vi "Get Encoders.vi"   [LabVIEW 2012]
uses:
  Robot Global Data.vi
types:
  T1 = typedef "WPI_EncoderDevRef.ctl" = cluster{"DevStatus":errorcluster, "EncoderIndex":T2, "CounterIndex":T3, "DistancePerCount":dbl, "Decoding Type":T4}
  T2 = typedef "FPGA_EncoderIdx.ctl" = enum8{"Enc 0", "Enc 1", "Enc 2", "Enc 3", "Invalid"}
  T3 = typedef "FPGA_CounterCtrSystemIndex.ctl" = enum8{"Ctr 0", "Ctr 1", "Ctr 2", "Ctr 3", "Ctr 4", "Ctr 5", "Ctr 6", "Ctr 7", "Invalid"}
  T4 = typedef "WPI_EncoderType.ctl" = enum16{"1x", "2x", "4x"}
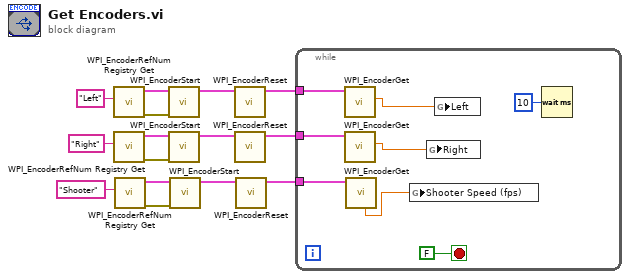
[diagram p0: block diagram]
diagram:
  n1 = call <vilib>:"WPI_EncoderRefNum Registry Get.vi"("refnum name"="Left") -> ("error out"=w15:errorcluster, "EncoderDevRef"=w14:T1)  [unwired: 9 in]
  n2 = call <vilib>:"WPI_EncoderRefNum Registry Get.vi"("refnum name"="Right") -> ("error out"=w10:errorcluster, "EncoderDevRef"=w9:T1)  [unwired: 9 in]
  n3 = call <vilib>:"WPI_EncoderRefNum Registry Get.vi"("refnum name"="Shooter") -> ("error out"=w5:errorcluster, "EncoderDevRef"=w4:T1)  [unwired: 9 in]
  n4 = call <vilib>:"WPI_EncoderStart.vi"("error in (no error)"=w15, "EncoderDevRef"=w14) -> ("EncoderDevRef"=w13:T1)  [unwired: 8 in, 1 out]
  n5 = call <vilib>:"WPI_EncoderStart.vi"("error in (no error)"=w10, "EncoderDevRef"=w9) -> ("EncoderDevRef"=w8:T1)  [unwired: 8 in, 1 out]
  n6 = call <vilib>:"WPI_EncoderStart.vi"("error in (no error)"=w5, "EncoderDevRef"=w4) -> ("EncoderDevRef"=w3:T1)  [unwired: 8 in, 1 out]
  n7 = call <vilib>:"WPI_EncoderReset.vi"("EncoderDevRef"=w13) -> ("EncoderDevRef"=w11:T1)  [unwired: 9 in, 1 out]
  n8 = call <vilib>:"WPI_EncoderReset.vi"("EncoderDevRef"=w8) -> ("EncoderDevRef"=w6:T1)  [unwired: 9 in, 1 out]
  n9 = call <vilib>:"WPI_EncoderReset.vi"("EncoderDevRef"=w3) -> ("EncoderDevRef"=w1:T1)  [unwired: 9 in, 1 out]
  n10 = while {
    tunnel: w11 -> [w23]
    tunnel: w6 -> [w22]
    tunnel: w1 -> [w21]
    stop <- FALSE stop-if-true
    n11 = call <vilib>:"WPI_EncoderGet.vi"("EncoderDevRef"=w23) -> ("Distance"=w18:dbl)  [unwired: 5 in, 5 out]
    n12 = call <vilib>:"WPI_EncoderGet.vi"("EncoderDevRef"=w22) -> ("Distance"=w17:dbl)  [unwired: 5 in, 5 out]
    n13 = call <vilib>:"WPI_EncoderGet.vi"("EncoderDevRef"=w21) -> ("Rate"=w19:dbl)  [unwired: 5 in, 5 out]
    n14 = global write "Robot Global Data.vi" "Shooter Speed (fps)"(w19) -> ()
    n15 = global write "Robot Global Data.vi" "Right"(w17) -> ()
    n16 = global write "Robot Global Data.vi" "Left"(w18) -> ()
    n17 = Wait (ms)(milliseconds to wait=u32 10) -> ()  [unwired: 1 out]
  }
